vi "File open.vi"(10 "file name":string) -> (0 "log":refnum<file>, 2 "cmd":string[](array[string]))   [LabVIEW 2018]
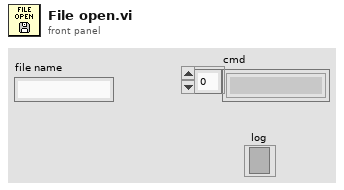
[diagram p1: front panel]
types:
  T1 = enum16{"open", "replace", "create", "open or create", "replace or create", "replace or create with confirmation"}
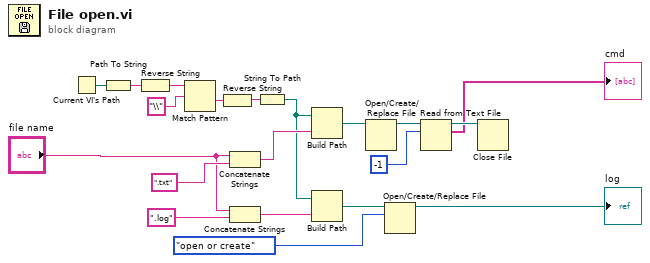
[diagram p0: block diagram]
diagram:
  n1 = Current VI's Path() -> (path=w17:path)
  n2 = Path To String(path=w17) -> (string=w16:string)
  n3 = Reverse String(1:w16) -> (0:w15:string)
  n4 = Match Pattern(string=w15, regular expression="\\") -> (after substring=w19:string)  [unwired: 1 in, 3 out]
  n5 = Reverse String(1:w19) -> (0:w18:string)
  n6 = Concatenate Strings("file name", ".txt" ("regular expression")) -> (w14:string)
  n7 = Concatenate Strings("file name", ".log" ("regular expression")) -> (w13:string)
  n8 = String To Path(string=w18) -> (path=w2:path)
  n9 = Build Path(base path=w2, name or relative path=w14) -> (appended path=w5:path)
  n10 = Build Path(base path=w2, name or relative path=w13) -> (appended path=w10:path)
  n11 = Open/Create/Replace File(file path (use dialog)=w5) -> (refnum out=w8:refnum<file>)  [unwired: 5 in, 2 out]
  n12 = Open/Create/Replace File(file path (use dialog)=w10, operation (0:open)=T1."open or create") -> (refnum out=→"log":refnum<file>)  [unwired: 4 in, 2 out]
  n13 = Read from Text File(file (use dialog)=w8, count=-1) -> (refnum out=w7:refnum<file>, text=→"cmd":string[])  [unwired: 2 in, 2 out]
  n14 = Close File(refnum=w7) -> ()  [unwired: 1 in, 2 out]
